vi "UpdateCoinArray.vi"(8 "error in (no error)":errorcluster, 10 "Coins Values":dbl[](array[numeric]), 11 "Coins in":refnum<class "Coins.lvclass">) -> (0 "error out":errorcluster, 3 "Coins out":refnum<class "Coins.lvclass">)   [LabVIEW 2020, in "Coins.lvlib" / "Coins.lvclass"]
uses:
  Coins.lvclass
  Coins.lvclass/Coins.ctl
  Write Coins Values.vi
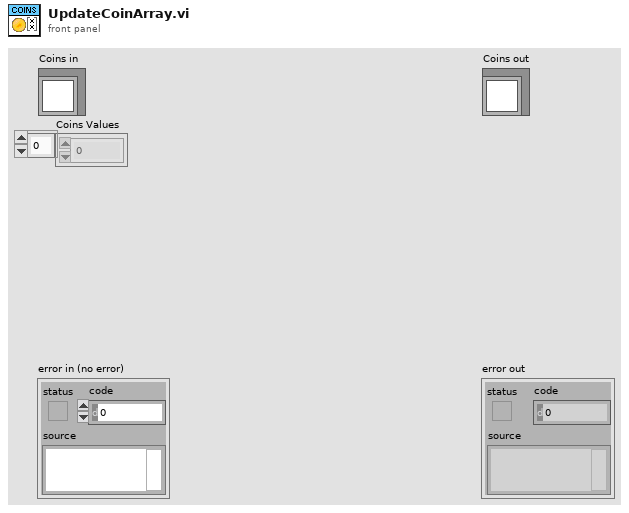
[diagram p1: front panel]
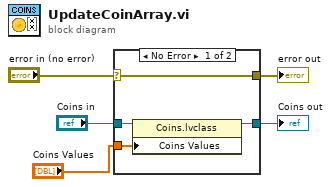
[diagram p0: block diagram]
diagram:
  n1 = case shown="No Error" "error in (no error)" {
    selector: "error in (no error)" -> [w8 w11]
    tunnel: [w8 w11] -> w4
    tunnel: [w7 w10] -> w2
    tunnel: "Coins in" -> [w9 w10]
    tunnel: "Coins Values" -> [w6 _]
    frame No Error {
      n2 = property class="Coins.lvclass"(reference=w9, "Coins Values"=w6) -> (reference out=w7:refnum<class "Coins.lvclass">)  [unwired: 1 in, 1 out]
    }
    frame Error {
    }
  }
  "error out" <- w4
  "Coins out" <- w2
